vi "SR830 Sweep Voltage and Record to file.vi"() -> ()   [LabVIEW 2018]
uses:
  <instrlib>/Stanford Research 830/Public/Data/Read (All Parameters).vi
  <instrlib>/Stanford Research 830/Stanford Research 830.lvlib
panel:
  in  "Time Constant":u16(ring)=8 items=["10 us", "30 us", "100 us", "300 us", "1 ms", "3 ms", "10 ms", "30 ms", "100 ms", "300 ms", "1 s", "3 s", "10 s", "30 s", "100 s", "300 s", "1 ks", "3 ks", "10 ks", "30 ks"]
  in  "File to save to":path
  out "Measured voltage (V, RMS)":dbl format="%#_6p"
  in  "Input coupling":u16(ring) items=["AC", "DC"]
  in  "Input connection":u16(ring) items=["Single-Ended Voltage", "Differential Voltage", "1 MOhm Current Gain", "100 MOhm Current Gain"]
  in  "Dynamic reserve":i16(ring)=2 items=["High Reserve"=0, "Normal"=1, "Low Noise"=2, "Auto Reserve"=-1]
  in  "Sensitivity":i16(ring)=12 items=["Auto Gain"=-1, "2 nV/fA"=0, "5 nV/fA"=1, "10 nV/fA"=2, "20 nV/fA"=3, "50 nV/fA"=4, "100 nV/fA"=5, "200 nV/fA"=6, "500 nV/fA"=7, "1 uV/pA"=8, "2 uV/pA"=9, "5 uV/pA"=10, "10 uV/pA"=11, "20 uV/pA"=12, "50 uV/pA"=13, "100 uV/pA"=14, "200 uV/pA"=15, "500 uV/pA"=16, "1 mV/nA"=17, "2 mV/nA"=18, "5 mV/nA"=19, "10 mV/nA"=20, "20 mV/nA"=21, "50 mV/nA"=22, "100 mV/nA"=23, "200 mV/nA"=24, "500 mV/mA"=25, "1 V/uA"=26]
  in  "VISA resource name of Stanford SR830":refnum<visa-resource-name>="GPIB0::9::INSTR"
  in  "Wait before measuring (s)":dbl=1.0 format="%#_6p"
  out "Step":dbl format="%^#_6e"
  out "Voltage (V)":dbl format="%#_6p"
  in  "Steps":dbl=5.0 format="%^#_6e"
  in  "Frequency (Hz)":dbl=866.0 format="%#_6p"
  in  "End voltage (V)":dbl=0.03 format="%#_6p"
  in  "Start voltage (V)":dbl=0.005 format="%#_6p"
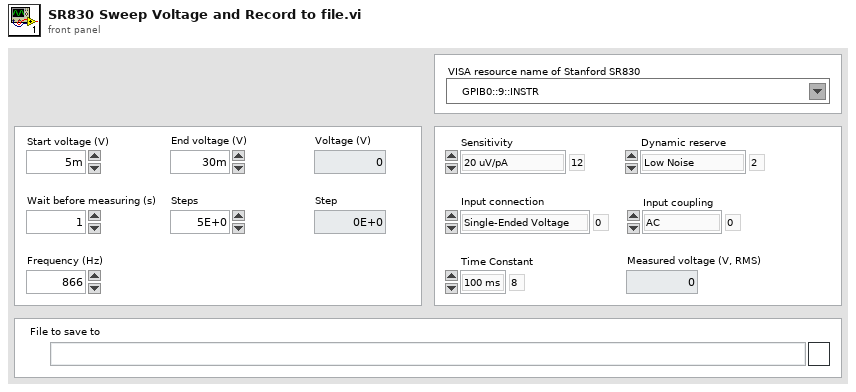
[diagram p1: front panel]
types:
  T1 = cluster{"X-Value":dbl, "Y-Value":dbl, "R-Value":dbl, "Theta-Value":dbl, "Aux In 1 Value":dbl, "Aux In 2 Value":dbl, "Aux In 3 Value":dbl, "Aux In 4 Value":dbl, "Reference Frequency":dbl, "Channel 1 Display":dbl, "Channel 2 Display":dbl}
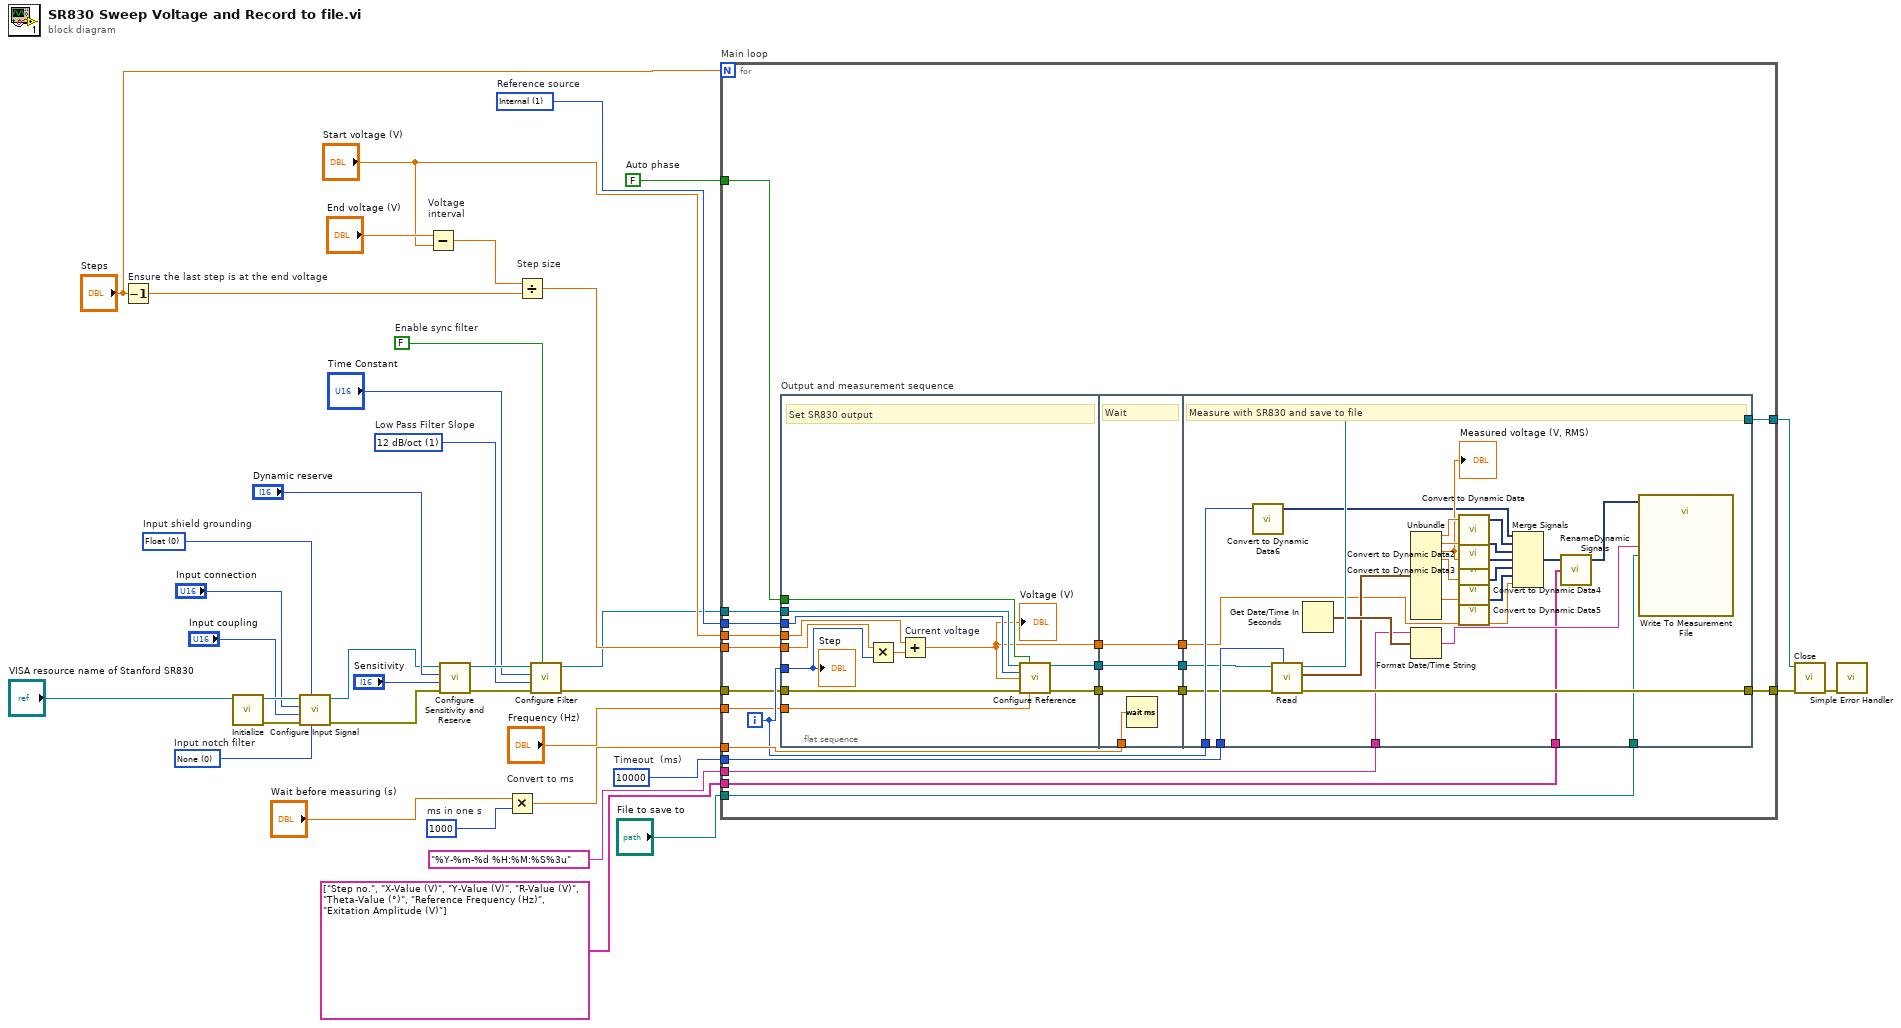
[diagram p0: block diagram]
diagram:
  w14 = u32 10000  # Timeout  (ms)
  w15 = u16 1 items=["6 dB/oct", "12 dB/oct", "18 db/oct", "24 dB/oct"]  # Low Pass Filter Slope
  w19 = FALSE  # Enable sync filter
  w7 = FALSE  # Auto phase
  w22 = u16 0 items=["None", "Line Notch", "2x Line Notch", "Both Notch Filters"]  # Input notch filter
  w6 = u16 1 items=["External", "Internal"]  # Reference source
  w26 = u16 0 items=["Float", "Ground"]  # Input shield grounding
  w31 = 1000  # ms in one s
  n1 = Decrement "Ensure the last step is at the end voltage"(x="Steps") -> (x-1=w29:dbl)
  n2 = call <instrlib>:"Initialize.vi"("VISA resource name"="VISA resource name of Stanford SR830") -> ("error out"=w23:errorcluster, "VISA resource name out"=w27:refnum<visa-resource-name>)  [unwired: 9 in]
  n3 = call <instrlib>:"Configure Input Signal.vi"("Input Notch Filter (0: None)"=w22, "Input Shield Grounding (0: Float)"=w26, "error in (no error)"=w23, "Input Coupling (0: AC)"="Input coupling", "Input Connection (0: Single-Ended Voltage)"="Input connection", "VISA resource name"=w27) -> ("error out"=w4:errorcluster, "VISA resource name out"=w5:refnum<visa-resource-name>)  [unwired: 4 in]
  n4 = Subtract "Voltage\ninterval"(x="End voltage (V)", y="Start voltage (V)") -> (x-y=w36:dbl)
  n5 = call <instrlib>:"Configure Sensitivity and Reserve.vi"("error in (no error)"=w4, "Sensitivity (-1: Auto gain)"="Sensitivity", "Dynamic Reserve (-1: Auto Reserve)"="Dynamic reserve", "VISA resource name"=w5) -> ("error out"=w17:errorcluster, "VISA resource name out"=w18:refnum<visa-resource-name>)  [unwired: 6 in]
  n6 = Multiply "Convert to ms"(x="Wait before measuring (s)", y=w31) -> (x*y=w33:dbl)
  n7 = Divide "Step size"(x=w36, y=w29) -> (x/y=w35:dbl)
  n8 = call <instrlib>:"Configure Filter.vi"("Enable Sync Filter (F: Disable)"=w19, "error in (no error)"=w17, "Low Pass Filter Slope (1: 12dB/oct)"=w15, "Time Constant (8: 100ms)"="Time Constant", "VISA resource name"=w18) -> ("error out"=w2:errorcluster, "VISA resource name out"=w3:refnum<visa-resource-name>)  [unwired: 5 in]
  n9 = for "Main loop" {
    N: "Steps" -> [_]
    tunnel: w35 -> [w58]
    tunnel: "Start voltage (V)" -> [w57]
    tunnel: w33 -> [w56]
    tunnel: "Frequency (Hz)" -> [w38]
    tunnel: w14 -> [w55]
    tunnel: [w54] -> w9
    tunnel: [w53] -> w8
    tunnel: "File to save to" -> [w52]
    tunnel: "%Y-%m-%d %H:%M:%S%3u" -> [w51]
    tunnel: string[] ["Step no.", "X-Value (V)", "Y-Value (V)", "R-Value (V)", "Theta-Value (°)", "Reference Frequency (Hz)", "Exitation Amplitude (V)"] -> [w50]
    tunnel: w7 -> [w48]
    tunnel: w6 -> [w47]
    tunnel: w3 -> [w46]
    tunnel: w2 -> [w45]
    i -> [w49]
    n10 = flat-sequence "Output and measurement sequence" {
      tunnel: w49 -> [w67]
      tunnel: w58 -> [w69]
      tunnel: w57 -> [w68]
      tunnel: w48 -> [w66]
      tunnel: w47 -> [w65]
      tunnel: w46 -> [w64]
      tunnel: w45 -> [w63]
      tunnel: [w62] -> w43
      tunnel: [w61] -> w41
      tunnel: [w60] -> w39
      tunnel: w38 -> [w59]
      tunnel: w56 -> [w74]
      tunnel: [w73] -> w44
      tunnel: w43 -> [w73]
      tunnel: [w72] -> w42
      tunnel: w41 -> [w72]
      tunnel: [w71] -> w40
      tunnel: w39 -> [w71]
      tunnel: w55 -> [w100]
      tunnel: [w99] -> w54
      tunnel: [w98] -> w53
      tunnel: w52 -> [w84]
      tunnel: w51 -> [w83]
      tunnel: w50 -> [w82]
      tunnel: w49 -> [w80]
      tunnel: w44 -> [w78]
      tunnel: w42 -> [w77]
      tunnel: w40 -> [w76]
      frame #0 {
        # "Set SR830 output"
        n11 = Multiply(x=w69, y=w67) -> (x*y=w70:dbl)
        n12 = Add "Current voltage"(x=w68, y=w70) -> (x+y=w60:dbl)
        "Voltage (V)" <- w60
        n13 = call <instrlib>:"Configure Reference.vi"("VISA resource name"=w64, "Auto Phase (T: Enabled)"=w66, "Reference Source (1: Internal)"=w65, "Sine Output Amplitude (1 V)"=w60, "error in (no error)"=w63, "Internal Reference Frequency (1000 Hz)"=w59) -> ("VISA resource name out"=w62:refnum<visa-resource-name>, "error out"=w61:errorcluster)  [unwired: 8 in]
        "Step" <- w67
      }
      frame #1 {
        # "Wait"
        n14 = Wait (ms)(milliseconds to wait=w74) -> ()  [unwired: 1 out]
      }
      frame #2 {
        # "Measure with SR830 and save to file"
        n15 = call "Convert to Dynamic Data6"("Double"=w80) -> ("Dynamic Data Type"=w79:dynamicdata)  [unwired: 3 in]
        n16 = call-poly <instrlib>:"Read.vi"("Timeout (10000 ms)"=w100, "error in (no error)"=w77, "VISA resource name"=w78) -> ("error out"=w98:errorcluster, "Parameter Values"=w86:T1, "VISA resource name out"=w99:refnum<visa-resource-name>)  [unwired: 6 in]
        n17 = Get Date/Time In Seconds() -> (seconds since 1Jan1904=w88:timestamp)
        n18 = Unbundle(w86) -> ("X-Value"=w96:dbl, "Y-Value"=w95:dbl, "R-Value"=w81:dbl, "Theta-Value"=w85:dbl, "Reference Frequency"=w75:dbl)  [unwired: 6 out]
        "Measured voltage (V, RMS)" <- w81
        n19 = Format Date/Time String(time format string (%c)=w83, seconds (now)=w88) -> (date/time string=w87:string)  [unwired: 1 in]
        n20 = call "Convert to Dynamic Data"("Double"=w96) -> ("Dynamic Data Type"=w89:dynamicdata)  [unwired: 3 in]
        n21 = call "Convert to Dynamic Data2"("Double"=w95) -> ("Dynamic Data Type"=w90:dynamicdata)  [unwired: 3 in]
        n22 = call "Convert to Dynamic Data3"("Double"=w81) -> ("Dynamic Data Type"=w91:dynamicdata)  [unwired: 3 in]
        n23 = call "Convert to Dynamic Data4"("Double"=w85) -> ("Dynamic Data Type"=w92:dynamicdata)  [unwired: 3 in]
        n24 = call "Convert to Dynamic Data5"("Double"=w75) -> ("Dynamic Data Type"=w93:dynamicdata)  [unwired: 3 in]
        n25 = Merge Signals(w79, w89, w90, w91, w92, w93, w76) -> (w94:dynamicdata)
        n26 = call "RenameDynamicSignals.vi"("New Signal Names"=w82, "Dynamic Data In"=w94) -> ("Dynamic Data Out"=w97:dynamicdata)  [unwired: 2 in, 1 out]
        n27 = call "Write To Measurement File"("Signals"=w97, "Filename"=w84, "Comment"=w87) -> ()  [unwired: 14 in, 3 out]
      }
    }
  }
  n28 = call <instrlib>:"Close.vi"("error in (no error)"=w8, "VISA resource name"=w9) -> ("error out"=w13:errorcluster)  [unwired: 9 in]
  n29 = call <vilib>:"Simple Error Handler.vi"("error in (no error)"=w13) -> ()  [unwired: 4 in, 5 out]
